vi "Get Variables.vi"(8 "error in (no error)":errorcluster, 11 "Message Popup in":refnum<class "Numeric Functions.lvclass">) -> (0 "error out":errorcluster, 2 "Variables":variant, 3 "Message Popup out":refnum<class "Numeric Functions.lvclass">)   [LabVIEW 2016, in "Numeric Functions.lvclass"]
uses:
  Numeric Functions.lvclass
  Numeric Functions.lvclass/Numeric Functions.ctl
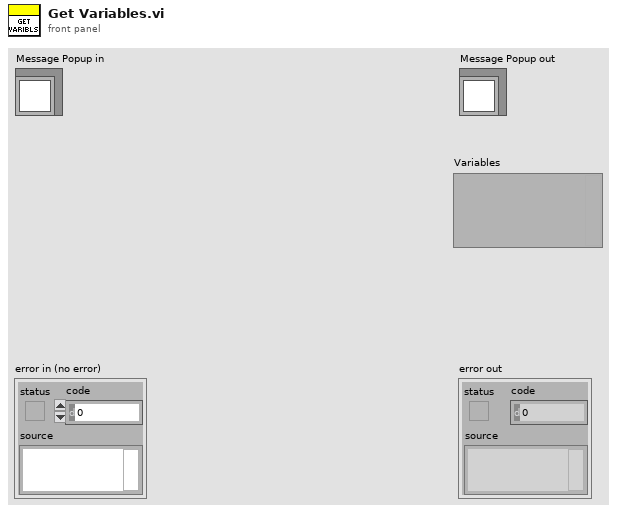
[diagram p1: front panel]
types:
  T1 = typedef "Arithmetic Operations.lvclass/Variables.ctl" = cluster{"Var1":dbl, "Var2":dbl}
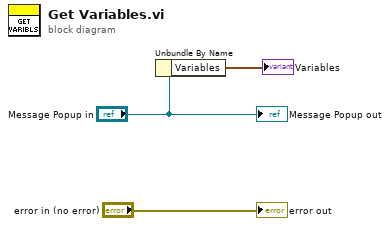
[diagram p0: block diagram]
diagram:
  n1 = Unbundle By Name("Message Popup in") -> ("Variables"=→"Variables":T1)
  "error out" <- "error in (no error)"
  "Message Popup out" <- "Message Popup in"
